vi "CAN refresh.vi"(8 "error in (no error)":errorcluster, 11 "CAN in":refnum<class "XNET_BS120x.lvclass">) -> (0 "error out":errorcluster, 3 "CAN out":refnum<class "XNET_BS120x.lvclass">)   [LabVIEW 2021, in "BS120x Driver.lvlib" / "XNET_BS120x.lvclass"]
uses:
  XNET_BS120x.lvclass
  XNET_BS120x.lvclass/XNET_BS120x.ctl
  _Private/Data Classes/XNET Data Class/XNET Data.lvclass/XNET Data.ctl
  _Private/Data Classes/XNET Data Class/Write XNET Array.vi
  <vilib>/xnet/xnet.llb/XNET Read (Frame CAN).vi
  _Private/Data Classes/XNET Data Class/XNET Data.lvclass
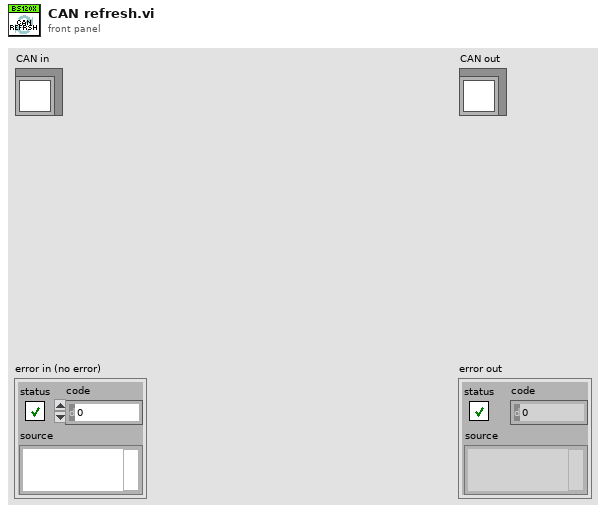
[diagram p1: front panel]
types:
  T1 = typedef "XNET Frame CAN.ctl" = cluster{"timestamp":timestamp, "payload":u8[], "identifier":u32, "type":T2, "extended?":bool, "echo?":bool}
  T2 = typedef "XNET Frame Type CAN.ctl" = u8
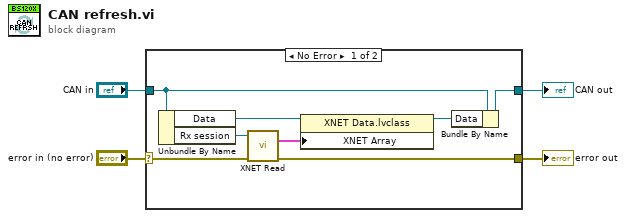
[diagram p0: block diagram]
diagram:
  n1 = case shown="No Error" "error in (no error)" {
    selector: "error in (no error)" -> [w8 w14]
    tunnel: [w7 w14] -> w3
    tunnel: [w9 w13] -> w1
    tunnel: "CAN in" -> [w11 w13]
    frame No Error {
      n2 = Unbundle By Name(w11) -> ("Data"=w6:refnum<class "XNET Data.lvclass">, "Rx session"=w5:refnum<k21>)
      n3 = call-poly <vilib>:"XNET Read.vi"("session in"=w5, "error in (no error)"=w8) -> ("data"=w12:T1[], "error out"=w7:errorcluster)  [unwired: 12 out]
      n4 = property class="XNET Data.lvclass"(reference=w6, "XNET Array"=w12) -> (reference out=w10:refnum<class "XNET Data.lvclass">)  [unwired: 1 in, 1 out]
      n5 = Bundle By Name(cluster=w11, "Data"=w10) -> (w9:refnum<class "XNET_BS120x.lvclass">)
    }
    frame Error {
    }
  }
  "error out" <- w3
  "CAN out" <- w1
